vi "Add Protection.vi"(8 "error in (no error)":errorcluster, 9 "Pad":bool, 10 "String in":string, 11 "LRC - HRZ Series in":refnum<class "LRC - HRZ Series.lvclass">) -> (0 "error out":errorcluster, 2 "String Out":string, 3 "LRC - HRZ Series out":refnum<class "LRC - HRZ Series.lvclass">)   [LabVIEW 2020, in "Protections.lvlib" / "LRC - HRZ Series.lvclass"]
uses:
  LRC - HRZ Series.lvclass
  LRC - HRZ Series.lvclass/LRC - HRZ Series.ctl
panel:
  out "resulting string":string
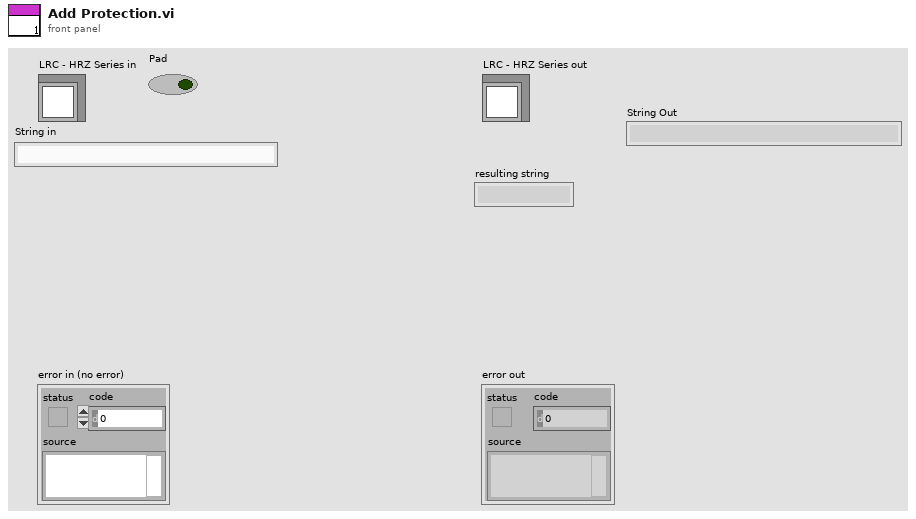
[diagram p1: front panel]
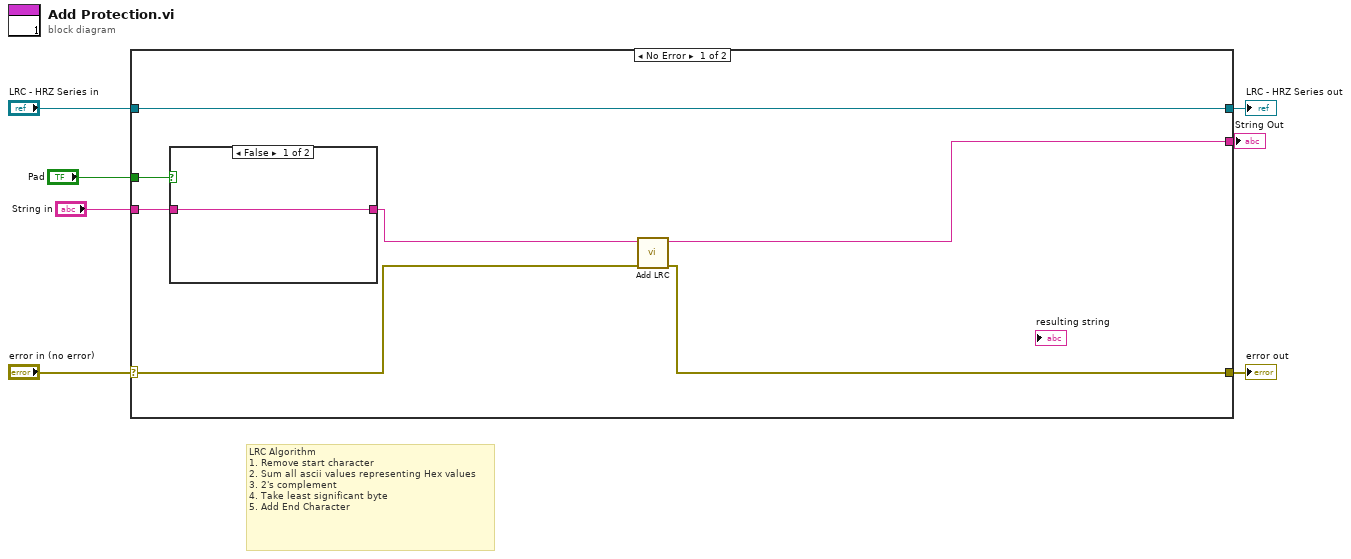
[diagram p0: block diagram]
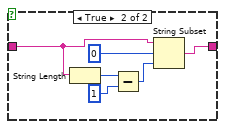
[diagram p2: hidden frame]
diagram:
  # "LRC Algorithm\n1. Remove start character\n2. Sum all ascii values representing Hex values \n3. 2's complement\n4. Take least significant byte\n5. Add End Character"
  n1 = case shown="No Error" "error in (no error)" {
    selector: "error in (no error)" -> [w10 w24]
    tunnel: [w9 w24] -> w6
    tunnel: [w14 w23] -> w4
    tunnel: "LRC - HRZ Series in" -> [w14 w23]
    tunnel: "Pad" -> [w13 _]
    tunnel: "String in" -> [w12 w22]
    tunnel: [w8 w22] -> w1
    frame No Error {
      n2 = case shown="False" w13 {
        tunnel: w12 -> [w15 w18]
        tunnel: [w15 w17] -> w11
        frame False {
        }
        frame True {
          n3 = String Length(string=w18) -> (length=w21:i32)
          n4 = Subtract(x=w21, y=1) -> (x-y=w19:i32)
          n5 = String Subset(string=w18, offset (0)=0, length (rest)=w19) -> (substring=w17:string)
        }
      }
      n6 = call "Add LRC.vi"("error in (no error)"=w10, "String in"=w11) -> ("error out"=w9:errorcluster, "String"=w8:string)  [unwired: 8 in]
    }
    frame Error {
    }
  }
  "error out" <- w6
  "LRC - HRZ Series out" <- w4
  "String Out" <- w1
